vi "Layer_Create or Substitute NI Layer.vi"(7 "New Picture":picture, 11 "All Layers":refnum<class "Layer.lvclass">[](array[class])) -> (3 "All Layers Out":refnum<class "Layer.lvclass">[](array[class]))   [LabVIEW 2021]
uses:
  vi.lib/LabVIEW Icon API/lv_icon/Classes/Layer/Layer.lvclass
  TypeDefs/Cluster_Layer Data.ctl
  vi.lib/LabVIEW Icon API/lv_icon/lv_icon.lvlib
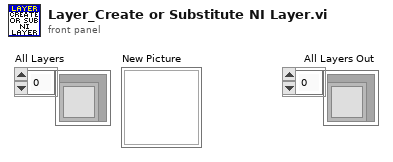
[diagram p1: front panel]
types:
  T1 = typedef "Cluster_Layer Data.ctl" = cluster{"LayerIcon":picture, "LayerName":string, "Opacity":u8, "Visibility?":bool}
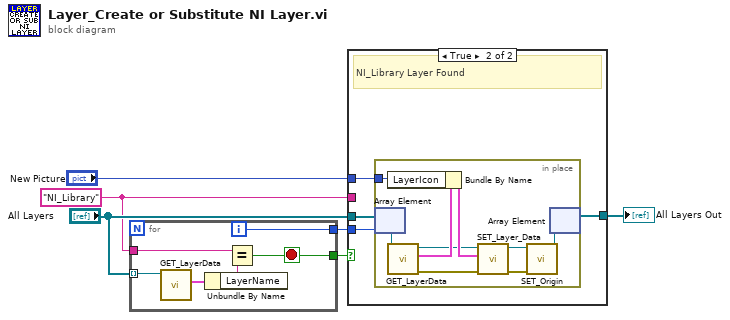
[diagram p0: block diagram]
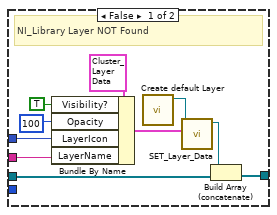
[diagram p2: hidden frame]
diagram:
  w4 = "NI_Library" ("LayerName")
  n1 = for {
    tunnel: "All Layers" -> [w12] mode=indexing
    tunnel: [w9] -> w3
    tunnel: [w8] -> w1
    tunnel: w4 -> [w7]
    i -> [w9]
    stop <- w8 stop-if-true
    n2 = call-dynamic "GET_LayerData.vi"("Layer.lvclass in"=w12) -> ("Data"=w11:T1)  [unwired: 1 in, 9 out]
    n3 = Unbundle By Name(w11) -> ("LayerName"=w10:string)
    n4 = Equal?(x=w7, y=w10) -> (x = y?=w8:bool)
  }
  n5 = case shown="True" w1 {
    tunnel: "All Layers" -> [w22 w25]
    tunnel: "New Picture" -> [w20 w26]
    tunnel: w3 -> [_ w24]
    tunnel: [w18 w23] -> w5
    tunnel: w4 -> [w15 _]
    frame False {
      # "NI_Library Layer NOT Found"
      n6 = Bundle By Name(cluster=T1 {"LayerIcon"=bytes[0], "LayerName"="", "Opacity"=0, "Visibility?"=FALSE} ("Data"), "Visibility?"=TRUE, "Opacity"=u8 100, "LayerIcon"=w20, "LayerName"=w15) -> (w19:T1)
      n7 = call "Create default Layer.vi"() -> ("Layer.lvclass out"=w17:refnum<class "Layer.lvclass">)  [unwired: 1 in, 10 out]
      n8 = call-dynamic "SET_Layer_Data.vi"("Data"=w19, "Layer.lvclass in"=w17) -> ("Layer.lvclass out"=w21:refnum<class "Layer.lvclass">)  [unwired: 2 in, 7 out]
      n9 = Build Array (concatenate)(w21, w22) -> (w18:refnum<class "Layer.lvclass">[])
    }
    frame True {
      # "NI_Library Layer Found"
      n10 = in-place {
        in-place-border: w26 -> [w32]
        n11 = in-place-array #1(w25, w24) -> (w28:refnum<class "Layer.lvclass">)
        n12 = call-dynamic "GET_LayerData.vi"("Layer.lvclass in"=w28) -> ("error out"=w29:errorcluster, "Data"=w33:T1, "Layer.lvclass out"=w30:refnum<class "Layer.lvclass">)  [unwired: 1 in, 7 out]
        n13 = Bundle By Name(cluster=w33, "LayerIcon"=w32) -> (w31:T1)
        n14 = call-dynamic "SET_Layer_Data.vi"("error in (no error)"=w29, "Data"=w31, "Layer.lvclass in"=w30) -> ("error out"=w34:errorcluster, "Layer.lvclass out"=w35:refnum<class "Layer.lvclass">)  [unwired: 1 in, 6 out]
        n15 = call-dynamic "SET_Origin.vi"("error in (no error)"=w34, "Layer.lvclass in"=w35) -> ("Layer.lvclass out"=w27:refnum<class "Layer.lvclass">)  [unwired: 1 in, 8 out]
        n16 = in-place-array #1(w27) -> (w23:refnum<class "Layer.lvclass">[])  [unwired: 1 out]
      }
    }
  }
  "All Layers Out" <- w5
